vi "Give.vi"(8 "error in (no error)":errorcluster caption="entrée d'erreur (pas d'erreur)", 11 "B en entrée":refnum<class "B.lvclass">) -> (0 "error out":errorcluster caption="sortie d'erreur", 3 "B en sortie":refnum<class "B.lvclass">)   [LabVIEW 2015, in "B.lvclass"]
uses:
  B.lvclass
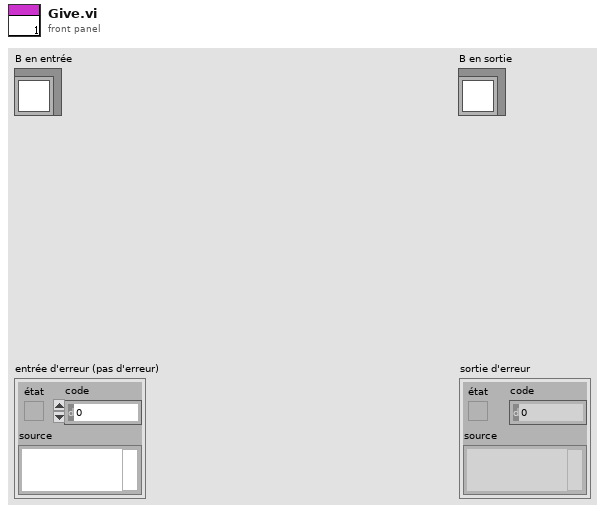
[diagram p1: front panel]
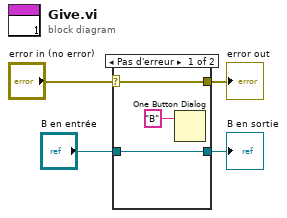
[diagram p0: block diagram]
diagram:
  n1 = case shown="Pas d'erreur" "error in (no error)" {
    selector: "error in (no error)" -> [w6 w9]
    tunnel: [w7 w8] -> w2
    tunnel: "B en entrée" -> [w7 w8]
    tunnel: [w6 w9] -> w1
    frame No Error {
      n2 = One Button Dialog(message="B") -> ()  [unwired: 1 in, 1 out]
    }
    frame Error {
    }
  }
  "error out" <- w1
  "B en sortie" <- w2
